vi "CMD_ETLSETUP.vi"(6 "Gantry in":refnum<class "Gantry.lvclass">, 8 "error in (no error)":errorcluster, 10 "Arguments":string[](array[string]), 11 "gScript Interpreter in":refnum<class "gScript Interpreter.lvclass">) -> (0 "error out":errorcluster, 3 "gScript Interpreter out":refnum<class "gScript Interpreter.lvclass">, 4 "Gantry out":refnum<class "Gantry.lvclass">)   [LabVIEW 2024, in "gScript Interpreter.lvclass"]
uses:
  gScript Interpreter.lvclass
  Shared Components/Gantry Class/Gantry.lvclass
  Shared Components/FlexWorktable/FlexWorktable.lvclass
  Shared Components/Database/ETL API.lvlib
panel:
  in  "Tab Control":enum32{"Module Setup", "Chip Placement"}(tab)
  out "module_4":T1
  out "module_3":T1
  out "module_2":T1
  out "module_1":T1
  in  "next":bool
  in  "n_modules":string(combo)="1" caption="Number of Modules"
  in  "module_id_1":string(combo) caption="Module ID"
  in  "module_id_2":string(combo) caption="Module ID"
  in  "module_id_3":string(combo) caption="Module ID"
  in  "module_id_4":string(combo) caption="Module ID"
  out "pos 16":string
  out "pos 15":string
  out "pos 14":string
  out "pos 13":string
  out "pos 12":string
  out "pos 11":string
  out "pos 10":string
  out "pos 9":string
  out "pos 8":string
  out "pos 7":string
  out "pos 6":string
  out "pos 5":string
  out "pos 4":string
  out "pos 3":string
  out "pos 2":string
  out "pos 1":string
  in  "finish":bool
  # "Position 1"
  # "Position 2"
  # "Position 3"
  # "Position 4"
  # "Stage the sub-assemblies according to the labels on the left. \nClick \"Finished\" when all chips & PCBs are staged."
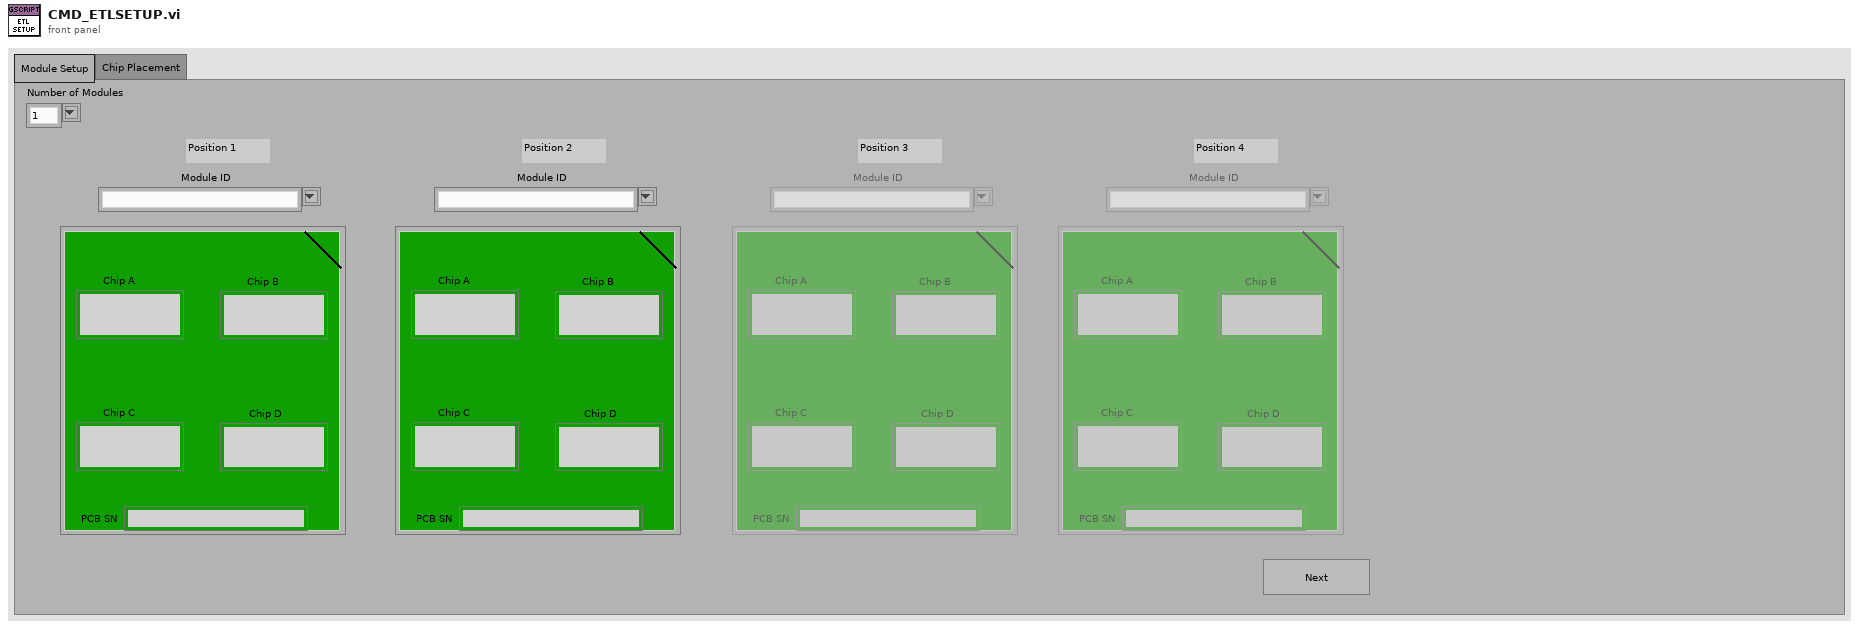
[diagram p1: front panel]
types:
  T1 = cluster{"Chip D":string, "Chip C":string, "Chip B":string, "Chip A":string, "PCB SN":string}
  T2 = enum8{"Enabled", "Disabled", "Disabled and Grayed Out"}
  T3 = typedef "ETL API.lvlib/ETL API Search Result.ctl" = cluster{"limit":i32, "total_results":i32, "results_ids":string[], "table":string}
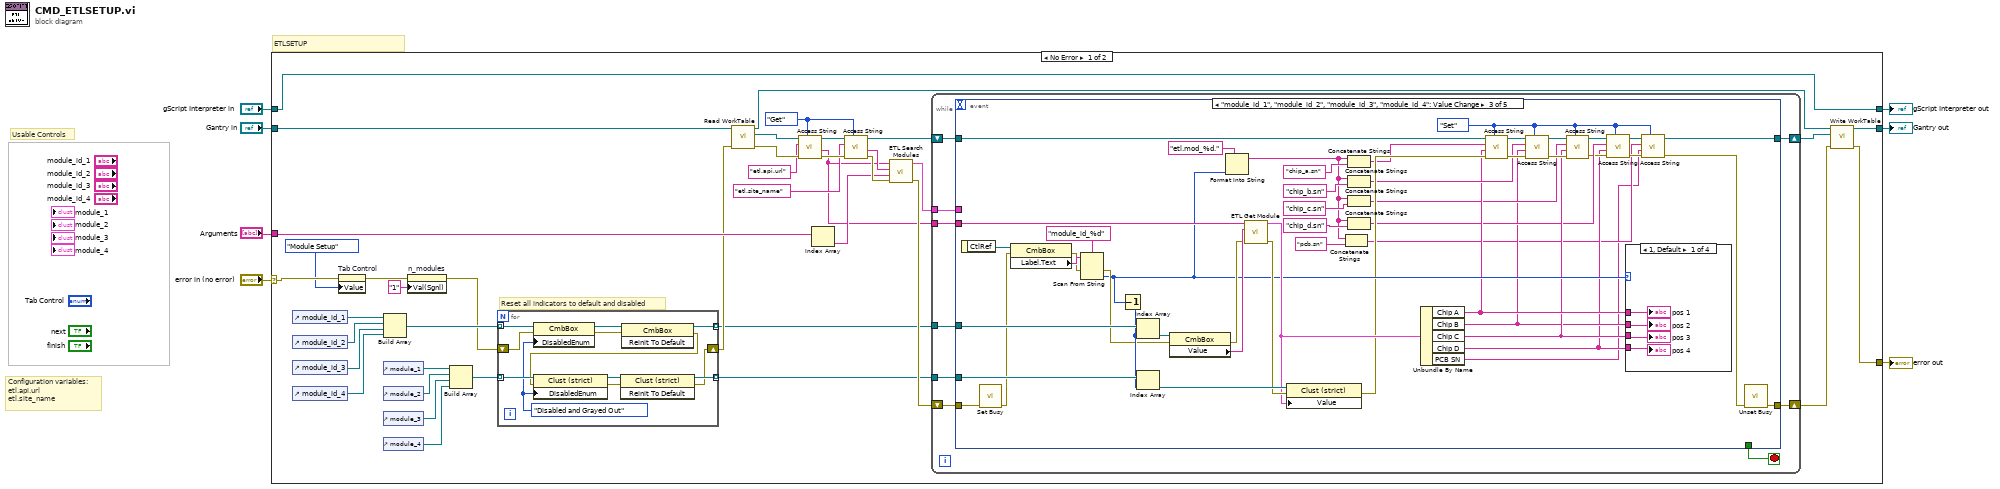
[diagram p0: block diagram]
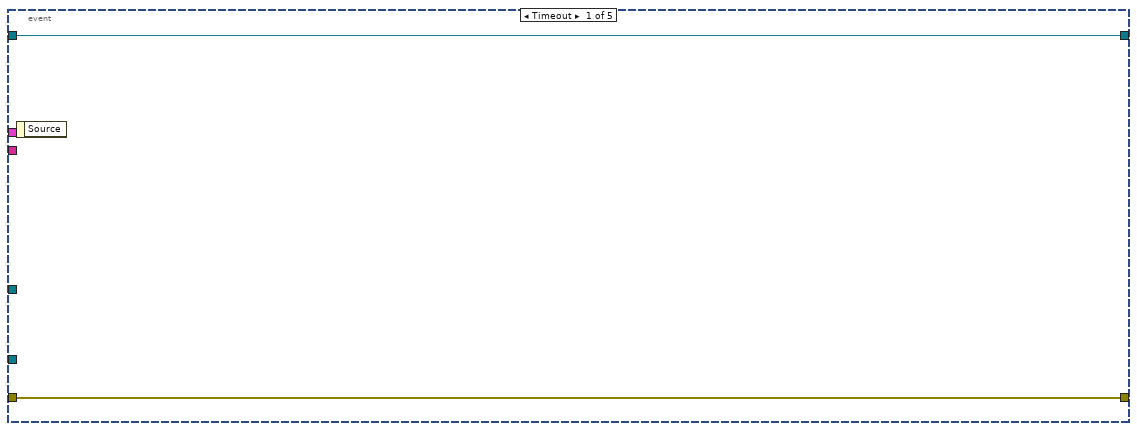
[diagram p2: hidden frame]
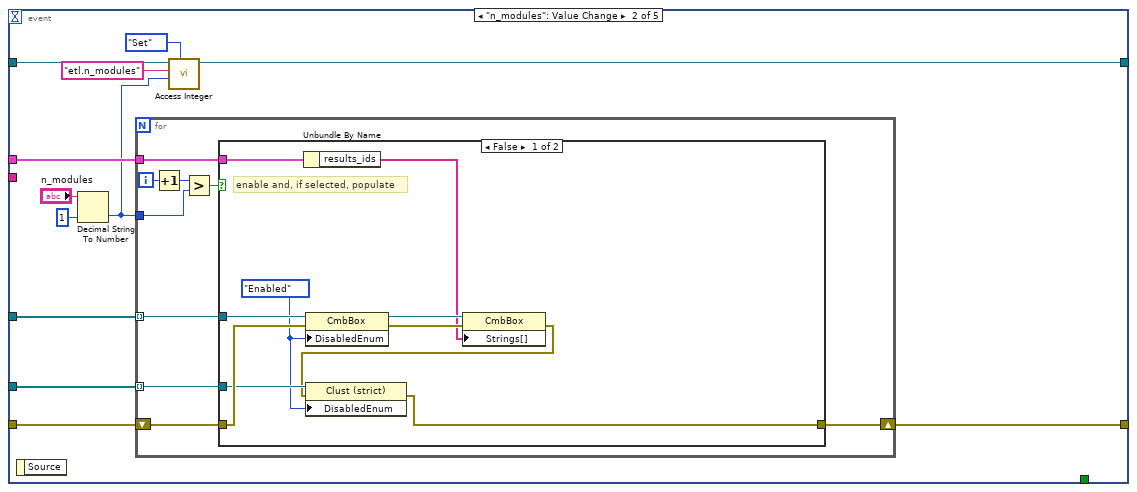
[diagram p3: hidden frame]
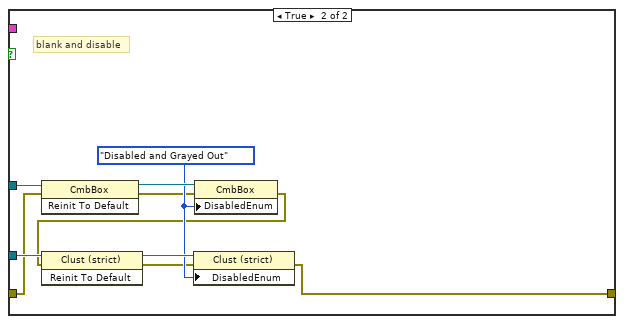
[diagram p4: hidden frame]
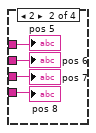
[diagram p5: hidden frame]
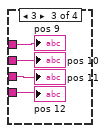
[diagram p6: hidden frame]
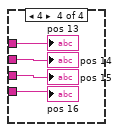
[diagram p7: hidden frame]
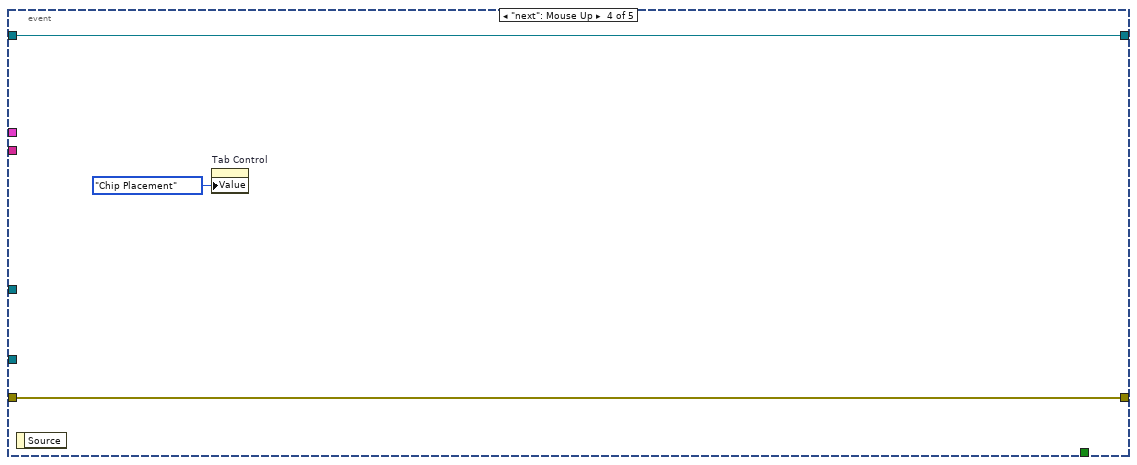
[diagram p8: hidden frame]
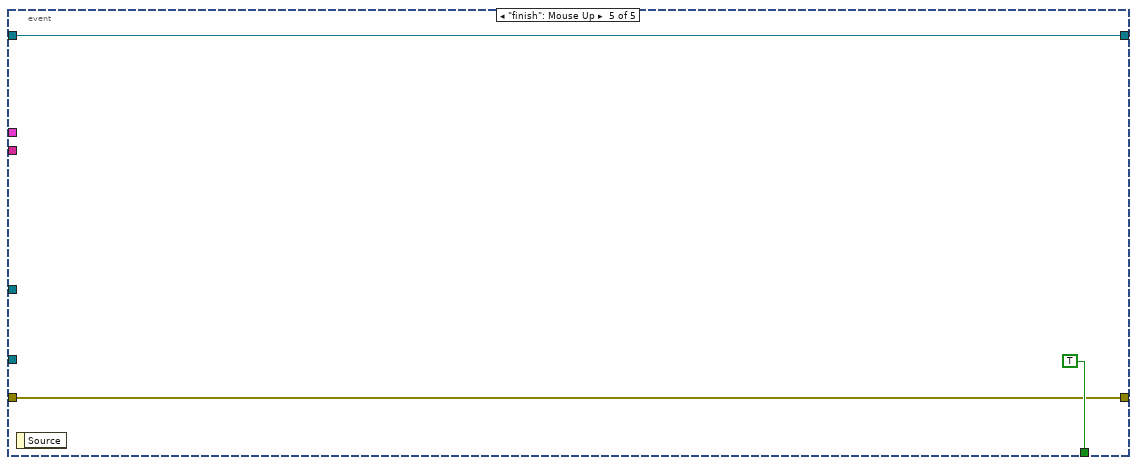
[diagram p9: hidden frame]
diagram:
  # "Configuration variables:\netl.api.url\netl.site_name"
  # "Usable Controls"
  # "ETLSETUP"
  n1 = case shown="No Error" "error in (no error)" {
    selector: "error in (no error)" -> [w16 w185]
    tunnel: [w8 w185] -> w6
    tunnel: [w10 w184] -> w4
    tunnel: "gScript Interpreter in" -> [w10 w184]
    tunnel: "Arguments" -> [w38 _]
    tunnel: "Gantry in" -> [w47 w183]
    tunnel: [w11 w183] -> w1
    frame No Error {
      w41 = enum16{"Get", "Set"}."Get" ("Get/Set")
      # "Reset all indicators to default and disabled"
      n2 = control-ref of="module_id_1"() -> (w35:refnum<vi>)
      n3 = control-ref of="module_id_2"() -> (w34:refnum<vi>)
      n4 = control-ref of="module_id_3"() -> (w33:refnum<vi>)
      n5 = control-ref of="module_id_4"() -> (w32:refnum<vi>)
      n6 = property on="Tab Control" class="TabCtl (strict)"(error in=w16, "Value"=enum32{"Module Setup", "Chip Placement"}."Module Setup" ("Tab Control")) -> (error out=w17:errorcluster)  [unwired: 1 in, 1 out]
      n7 = control-ref of="module_1"() -> (w31:refnum<vi>)
      n8 = control-ref of="module_2"() -> (w30:refnum<vi>)
      n9 = control-ref of="module_3"() -> (w29:refnum<vi>)
      n10 = control-ref of="module_4"() -> (w28:refnum<vi>)
      n11 = Build Array(w35, w34, w33, w32) -> (w25:refnum<vi>[])
      n12 = property on="n_modules" class="CmbBox"(error in=w17, "Val(Sgnl)"="1" ("Value (Signaling)")) -> (error out=w23:errorcluster)  [unwired: 1 in, 1 out]
      n13 = Build Array(w31, w30, w29, w28) -> (w24:refnum<vi>[])
      n14 = for {
        tunnel: w25 -> [w59] mode=indexing
        tunnel: w24 -> [w58] mode=indexing
        shift-right: [w48] -> w22
        shift-left: w23 -> [w56]
        tunnel: [w52] -> w21 mode=indexing
        tunnel: [w51] -> w20 mode=indexing
        w57 = T2."Disabled and Grayed Out" ("Disabled")
        n15 = property class="CmbBox"(reference=w59, error in=w56, "DisabledEnum"=w57) -> (reference out=w55:refnum<vi>, error out=w53:errorcluster)
        n16 = invoke class="CmbBox" method="Reinit To Default"(reference=w55, error in=w53) -> (reference out=w52:refnum<vi>, error out=w50:errorcluster)  [unwired: 1 in, 1 out]
        n17 = property class="Clust (strict)"(reference=w58, error in=w50, "DisabledEnum"=w57) -> (reference out=w54:refnum<vi>, error out=w49:errorcluster)
        n18 = invoke class="Clust (strict)" method="Reinit To Default"(reference=w54, error in=w49) -> (reference out=w51:refnum<vi>, error out=w48:errorcluster)  [unwired: 1 in, 1 out]
      }
      n19 = call-dynamic "Read WorkTable.vi"("error in"=w22, "Gantry Class in"=w47) -> ("error out"=w45:errorcluster, "Worktable"=w46:refnum<class "FlexWorktable.lvclass">, "Gantry Class out"=w12:refnum<class "Gantry.lvclass">)  [unwired: 7 in]
      n20 = call-dynamic "Access String.vi"("Get/Set"=w41, "error in (no error)"=w45, "Key"="etl.api.url", "FlexWorktable in"=w46) -> ("error out"=w43:errorcluster, "Value out"=w18:string, "FlexWorktable out"=w44:refnum<class "FlexWorktable.lvclass">)  [unwired: 5 in]
      n21 = Index Array(array=w38) -> (element=w37:string)  [unwired: 1 in]
      n22 = call-dynamic "Access String.vi"("Get/Set"=w41, "error in (no error)"=w43, "Key"="etl.site_name", "FlexWorktable in"=w44) -> ("error out"=w40:errorcluster, "Value out"=w39:string, "FlexWorktable out"=w14:refnum<class "FlexWorktable.lvclass">)  [unwired: 5 in]
      n23 = call "ETL Search Modules.vi"("error in (no error)"=w40, "Module Type"=w37, "Site Name"=w39, "Base URL"=w18) -> ("error out"=w27:errorcluster, "Search Result"=w36:T3)  [unwired: 6 in]
      n24 = while {
        tunnel: w36 -> [w68]
        tunnel: w21 -> [w66]
        tunnel: w20 -> [w65]
        shift-right: [w63] -> w9
        shift-left: w27 -> [w64]
        tunnel: w18 -> [w62]
        shift-right: [w60] -> w13
        shift-left: w14 -> [w61]
        stop <- w67 stop-if-true
        n25 = event shown="[2] \"module_id_1\", \"module_id_2\", \"module_id_3\", \"module_id_4\": Value Change" {
          selector: _ -> [_ _ _ _ _]
          dyn-events: _ -> [_ _ _ _ _]
          timeout: _ -> [_ _ _ _ _]
          tunnel: w68 -> [_ w80 _ _ _]
          tunnel: [_ _ _ _ TRUE] -> w67
          tunnel: w66 -> [_ w82 w159 _ _]
          tunnel: w65 -> [_ w81 w158 _ _]
          tunnel: w64 -> [w70 w79 w146 w178 w181]
          tunnel: [w70 w78 w144 w178 w181] -> w63
          tunnel: w62 -> [_ _ w160 _ _]
          tunnel: w61 -> [w69 w77 w131 w177 w180]
          tunnel: [w69 w71 w114 w177 w180] -> w60
          event Timeout {
            n26 = event-data() -> ()  [unwired: 1 in, 1 out]
          }
          event "n_modules": Value Change {
            n27 = event-data() -> ()  [unwired: 1 in, 1 out]
            n28 = Decimal String To Number(string="n_modules", default (0L)=1 ("default (0 I32)")) -> (number=w72:i32)  [unwired: 1 in, 1 out]
            n29 = for {
              tunnel: w82 -> [w88] mode=indexing
              tunnel: w81 -> [w87] mode=indexing
              tunnel: w80 -> [w84]
              shift-right: [w85] -> w78
              shift-left: w79 -> [w86]
              tunnel: w72 -> [w83]
              i -> [w91]
              n30 = Increment(x=w91) -> (x+1=w90:i32)
              n31 = Greater?(x=w90, y=w83) -> (0:w89:bool)
              n32 = case shown="False" w89 {
                tunnel: w88 -> [w101 w111]
                tunnel: w87 -> [w99 w110]
                tunnel: w86 -> [w100 w103]
                tunnel: [w97 w102] -> w85
                tunnel: w84 -> [w96 _]
                frame False {
                  w98 = T2."Enabled" ("Disabled")
                  # "enable and, if selected, populate"
                  n33 = Unbundle By Name(w96) -> ("results_ids"=w93:string[])
                  n34 = property class="CmbBox"(reference=w101, error in=w100, "DisabledEnum"=w98) -> (reference out=w95:refnum<vi>, error out=w94:errorcluster)
                  n35 = property class="CmbBox"(reference=w95, error in=w94, "Strings[]"=w93) -> (error out=w92:errorcluster)  [unwired: 1 out]
                  n36 = property class="Clust (strict)"(reference=w99, error in=w92, "DisabledEnum"=w98) -> (error out=w97:errorcluster)  [unwired: 1 out]
                }
                frame True {
                  w107 = T2."Disabled and Grayed Out" ("Disabled")
                  # "blank and disable"
                  n37 = invoke class="CmbBox" method="Reinit To Default"(reference=w111, error in=w103) -> (reference out=w109:refnum<vi>, error out=w106:errorcluster)  [unwired: 1 in, 1 out]
                  n38 = property class="CmbBox"(reference=w109, error in=w106, "DisabledEnum"=w107) -> (error out=w105:errorcluster)  [unwired: 1 out]
                  n39 = invoke class="Clust (strict)" method="Reinit To Default"(reference=w110, error in=w105) -> (reference out=w108:refnum<vi>, error out=w104:errorcluster)  [unwired: 1 in, 1 out]
                  n40 = property class="Clust (strict)"(reference=w108, error in=w104, "DisabledEnum"=w107) -> (error out=w102:errorcluster)  [unwired: 1 out]
                }
              }
            }
            n41 = call-dynamic "Access Integer.vi"("Get/Set"=enum16{"Get", "Set"}."Set", "Value in"=w72, "Key"="etl.n_modules", "FlexWorktable in"=w77) -> ("FlexWorktable out"=w71:refnum<class "FlexWorktable.lvclass">)  [unwired: 5 in, 2 out]
          }
          event "module_id_1", "module_id_2", "module_id_3", "module_id_4": Value Change {
            w115 = enum16{"Get", "Set"}."Set" ("Get/Set")
            n42 = event-data() -> ("CtlRef"=w154:refnum<vi>)  [unwired: 1 in]
            n43 = call <vilib>:"Set Busy.vi"("error in (no error)"=w146) -> ("error out"=w145:errorcluster)  [unwired: 9 in, 1 out]
            n44 = property class="CmbBox"(reference=w154, error in=w145) -> (error out=w151:errorcluster, "Label.Text"=w153:string)  [unwired: 1 out]
            n45 = Scan From String(format string="module_id_%d", input string=w153, error in=w151) -> (error out=w149:errorcluster, output 1=w141:i32)  [unwired: 2 in, 2 out]
            n46 = Decrement(x=w141) -> (x-1=w150:i32)
            n47 = Index Array(array=w159, index=w150) -> (element=w157:refnum<vi>)
            n48 = Index Array(array=w158, index=w150) -> (element=w148:refnum<vi>)
            n49 = property class="CmbBox"(reference=w157, error in=w149) -> (error out=w155:errorcluster, "Value"=w156:string)  [unwired: 1 out]
            n50 = Format Into String(format string="etl.mod_%d.", w141) -> (resulting string=w119:string)  [unwired: 2 in, 1 out]
            n51 = call "ETL Get Module.vi"("error in (no error)"=w155, "Module SN"=w156, "Base URL"=w160) -> ("error out"=w147:errorcluster, "Module Components"=w143:T1)  [unwired: 7 in]
            n52 = property class="Clust (strict)"(reference=w148, error in=w147, "Value"=w143) -> (error out=w130:errorcluster)  [unwired: 1 out]
            n53 = Concatenate Strings(w119, "pcb.sn") -> (w113:string)
            n54 = Concatenate Strings(w119, "chip_a.sn") -> (w129:string)
            n55 = Concatenate Strings(w119, "chip_b.sn") -> (w128:string)
            n56 = Concatenate Strings(w119, "chip_c.sn") -> (w126:string)
            n57 = Concatenate Strings(w119, "chip_d.sn") -> (w124:string)
            n58 = Unbundle By Name(w143) -> ("Chip A"=w127:string, "Chip B"=w123:string, "Chip C"=w125:string, "Chip D"=w121:string, "PCB SN"=w112:string)
            n59 = call-dynamic "Access String.vi"("Get/Set"=w115, "error in (no error)"=w130, "Value in"=w127, "Key"=w129, "FlexWorktable in"=w131) -> ("error out"=w136:errorcluster, "FlexWorktable out"=w134:refnum<class "FlexWorktable.lvclass">)  [unwired: 4 in, 1 out]
            n60 = call-dynamic "Access String.vi"("Get/Set"=w115, "error in (no error)"=w136, "Value in"=w123, "Key"=w128, "FlexWorktable in"=w134) -> ("error out"=w135:errorcluster, "FlexWorktable out"=w133:refnum<class "FlexWorktable.lvclass">)  [unwired: 4 in, 1 out]
            n61 = call-dynamic "Access String.vi"("Get/Set"=w115, "error in (no error)"=w135, "Value in"=w125, "Key"=w126, "FlexWorktable in"=w133) -> ("error out"=w122:errorcluster, "FlexWorktable out"=w132:refnum<class "FlexWorktable.lvclass">)  [unwired: 4 in, 1 out]
            n62 = call-dynamic "Access String.vi"("Get/Set"=w115, "error in (no error)"=w122, "Value in"=w121, "Key"=w124, "FlexWorktable in"=w132) -> ("error out"=w118:errorcluster, "FlexWorktable out"=w116:refnum<class "FlexWorktable.lvclass">)  [unwired: 4 in, 1 out]
            n63 = case shown="1, Default" w141 {
              tunnel: w127 -> [w164 w168 w172 w176]
              tunnel: w123 -> [w163 w167 w171 w175]
              tunnel: w125 -> [w162 w166 w170 w174]
              tunnel: w121 -> [w161 w165 w169 w173]
              frame 1, Default {
                "pos 1" <- w164
                "pos 2" <- w163
                "pos 3" <- w162
                "pos 4" <- w161
              }
              frame 2 {
                "pos 5" <- w168
                "pos 6" <- w167
                "pos 7" <- w166
                "pos 8" <- w165
              }
              frame 3 {
                "pos 9" <- w172
                "pos 10" <- w171
                "pos 11" <- w170
                "pos 12" <- w169
              }
              frame 4 {
                "pos 13" <- w176
                "pos 14" <- w175
                "pos 15" <- w174
                "pos 16" <- w173
              }
            }
            n64 = call-dynamic "Access String.vi"("Get/Set"=w115, "error in (no error)"=w118, "Value in"=w112, "Key"=w113, "FlexWorktable in"=w116) -> ("error out"=w117:errorcluster, "FlexWorktable out"=w114:refnum<class "FlexWorktable.lvclass">)  [unwired: 4 in, 1 out]
            n65 = call <vilib>:"Unset Busy.vi"("error in (no error)"=w117) -> ("error out"=w144:errorcluster)  [unwired: 10 in]
          }
          event "next": Mouse Up {
            n66 = event-data() -> ()  [unwired: 1 in, 1 out]
            n67 = property on="Tab Control" class="TabCtl (strict)"("Value"=enum32{"Module Setup", "Chip Placement"}."Chip Placement" ("Tab Control")) -> ()  [unwired: 2 in, 2 out]
          }
          event "finish": Mouse Up {
            n68 = event-data() -> ()  [unwired: 1 in, 1 out]
          }
        }
      }
      n69 = call-dynamic "Write WorkTable.vi"("error in (no error)"=w9, "FlexWorktable"=w13, "Gantry Class in"=w12) -> ("error out"=w8:errorcluster, "Gantry Class out"=w11:refnum<class "Gantry.lvclass">)  [unwired: 7 in]
    }
    frame Error {
    }
  }
  "error out" <- w6
  "gScript Interpreter out" <- w4
  "Gantry out" <- w1
